vi "Check if configuration files exist.vi"(8 "error in (no error)":errorcluster, 11 "TemplateBase in":refnum<class "Cobolt.lvclass">=refnum) -> (0 "error out":errorcluster, 2 "configuration file exists?":bool, 3 "TemplateBase out":refnum<class "Cobolt.lvclass">)   [LabVIEW 2012, in "Cobolt.lvclass"]
doc: "Checks whether all required configuration files for the component exist."
uses:
  Cobolt.lvclass
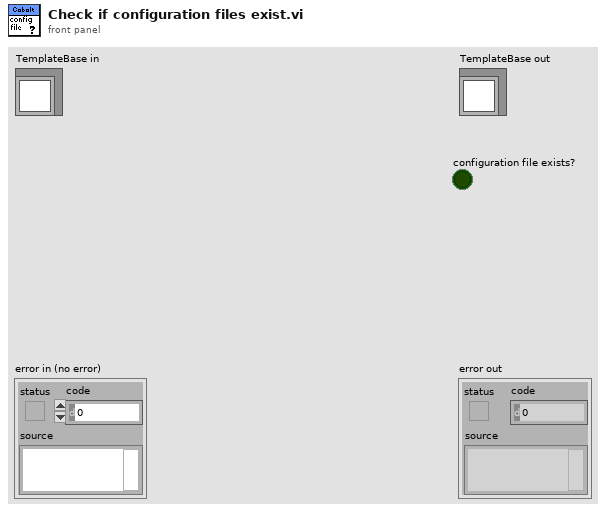
[diagram p1: front panel]
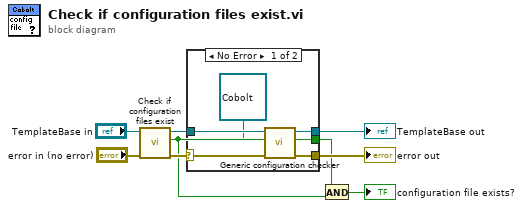
[diagram p0: block diagram]
diagram:
  n1 = call-parent "Check if configuration files exist.vi"("error in (no error)"="error in (no error)", "MurmexBase in"="TemplateBase in") -> ("error out"=w6:errorcluster, "configuration file exists?"=w2:bool, "MurmexBase out"=w5:refnum<class "Cobolt.lvclass">)  [unwired: 7 in]
  n2 = case shown="No Error" w6 {
    selector: w6 -> [w14 w16]
    tunnel: [w12 w16] -> w4
    tunnel: [w10 w15] -> w3
    tunnel: w5 -> [w13 w15]
    tunnel: [w11 _] -> _
    frame No Error {
      n3 = call "Generic configuration checker.vi"("error in (no error)"=w14, "inheritance level"=refnum<class "Cobolt.lvclass"> refnum ("Template.lvclass"), "Murmex in"=w13) -> ("error out"=w12:errorcluster, "configuration file exists?"=w11:bool, "Murmex out"=w10:refnum<class "Cobolt.lvclass">)  [unwired: 6 in]
    }
    frame Error {
    }
  }
  "error out" <- w4
  "TemplateBase out" <- w3
  n4 = And(x=w2, y=w2) -> (x .and. y?=→"configuration file exists?":bool)
